vi "Dispense FN - ON - State Status (SubVI).vi"(0 "Values IN":T1 {"Drain Time (s)" format="%.2f"; "Drain Rate (g/sec)" format="%.2f"}, 1 "Settings":T2={"ON Settings"={"Enable Dynamic Setpoint?"=TRUE, "Enable Dynamic Dispense Time?"=TRUE, "Enable Drain Rate Functions"=TRUE, "Dispense Sample Time (s)"=0.5, "Dispense Slope Ave"=0, "ON Timeout (sec)"=600.0, "1st Setpoint (% of Target)"=0.0, "2nd Setpoint (% of Target)"=0.0, "3rd Setpoint (% of Target)"=0.0, "Measure Dispense Delay (sec)"=0.0, "Settle Slope Sample Time (s)"=0.0}, "OFF Settings"={"Drain Sample Time (s)"=0.5, "Drain Rate Ave Size"=5, "Drain Rate Limits (± g/sec)"=10.0, "Level Slope Range (± g/sec)"=0.25, "OFF Timeout (sec)"=0.0, "Near SP Slope Level (± g/sec)"=0.01, "Near Setpoint Threshold (%)"=95.0}, "Overshoot Settings"={"Time Limit (s)"=60.0, "Container MAX (g)"=1500.0, "Max FILL Slope (+/- g/sec)"=10.0, "% Overshot to Enable (>)"=0.25}, "FILL Timeout (s)"=300.0, "Full Settle Time (s)"=3.0, "Pre-Hydrate \nSpray Time (s)"=10.0, "Pre-Hydrate \nWait Time (s)"=30.0}, 3 "Dynamic SP Valid?":bool, 4 "Enable Dispense Measure?":bool) -> (14 "Values OUT":T1, 16 "OFF Signal":bool, 17 "Dispense Timeout?":bool, 18 "Complete":bool)   [LabVIEW 2012]
panel:
  out "Time Setpoint (Un-used)":dbl
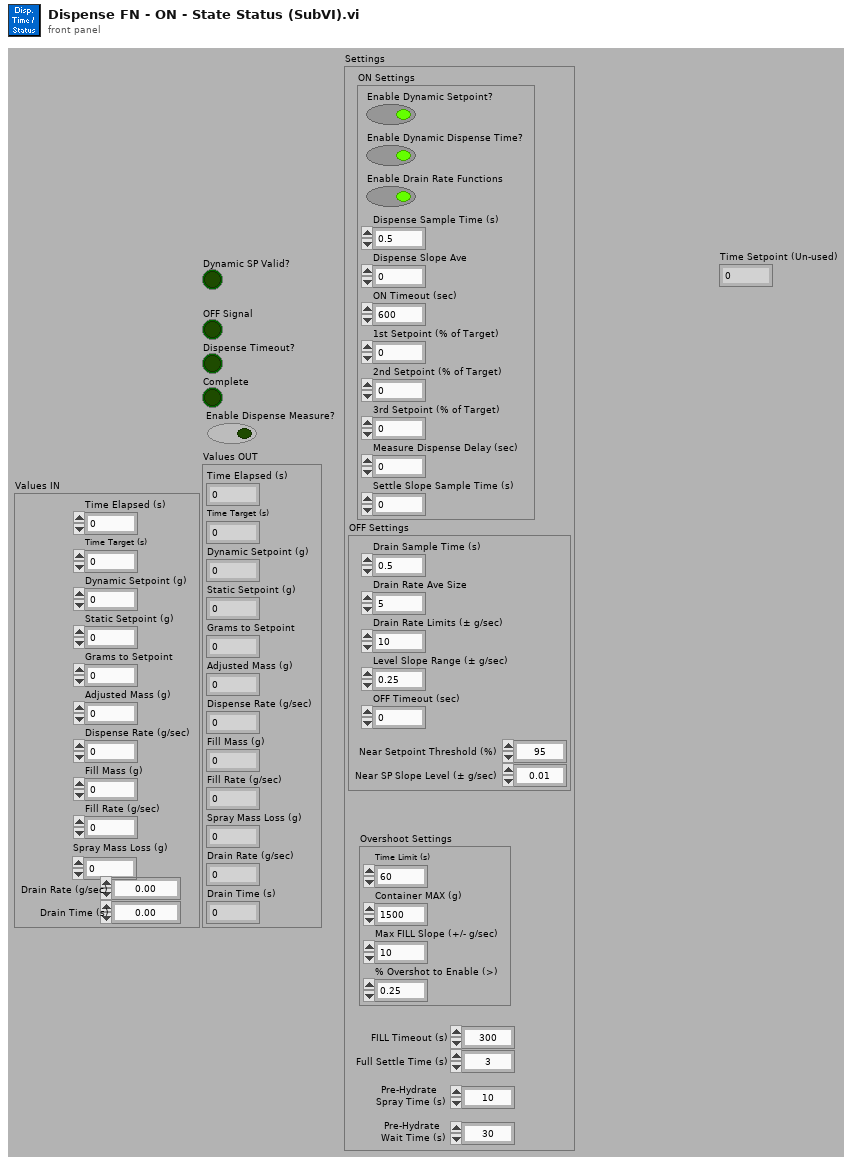
[diagram p1: front panel]
types:
  T1 = cluster{"Time Elapsed (s)":dbl, "Time Target (s)":dbl, "Dynamic Setpoint (g)":dbl, "Static Setpoint (g)":dbl, "Grams to Setpoint":dbl, "Adjusted Mass (g)":dbl, "Dispense Rate (g/sec)":dbl, "Fill Mass (g)":dbl, "Fill Rate (g/sec)":dbl, "Spray Mass Loss (g)":dbl, "Drain Rate (g/sec)":dbl, "Drain Time (s)":dbl}
  T2 = cluster{"ON Settings":cluster{"Enable Dynamic Setpoint?":bool, "Enable Dynamic Dispense Time?":bool, "Enable Drain Rate Functions":bool, "Dispense Sample Time (s)":dbl, "Dispense Slope Ave":i32, "ON Timeout (sec)":dbl, "1st Setpoint (% of Target)":dbl, "2nd Setpoint (% of Target)":dbl, "3rd Setpoint (% of Target)":dbl, "Measure Dispense Delay (sec)":dbl, "Settle Slope Sample Time (s)":dbl}, "OFF Settings":cluster{"Drain Sample Time (s)":dbl, "Drain Rate Ave Size":i32, "Drain Rate Limits (± g/sec)":dbl, "Level Slope Range (± g/sec)":dbl, "OFF Timeout (sec)":dbl, "Near SP Slope Level (± g/sec)":dbl, "Near Setpoint Threshold (%)":dbl}, "Overshoot Settings":cluster{"Time Limit (s)":dbl, "Container MAX (g)":dbl, "Max FILL Slope (+/- g/sec)":dbl, "% Overshot to Enable (>)":dbl}, "FILL Timeout (s)":dbl, "Full Settle Time (s)":dbl, "Pre-Hydrate \nSpray Time (s)":dbl, "Pre-Hydrate \nWait Time (s)":dbl}
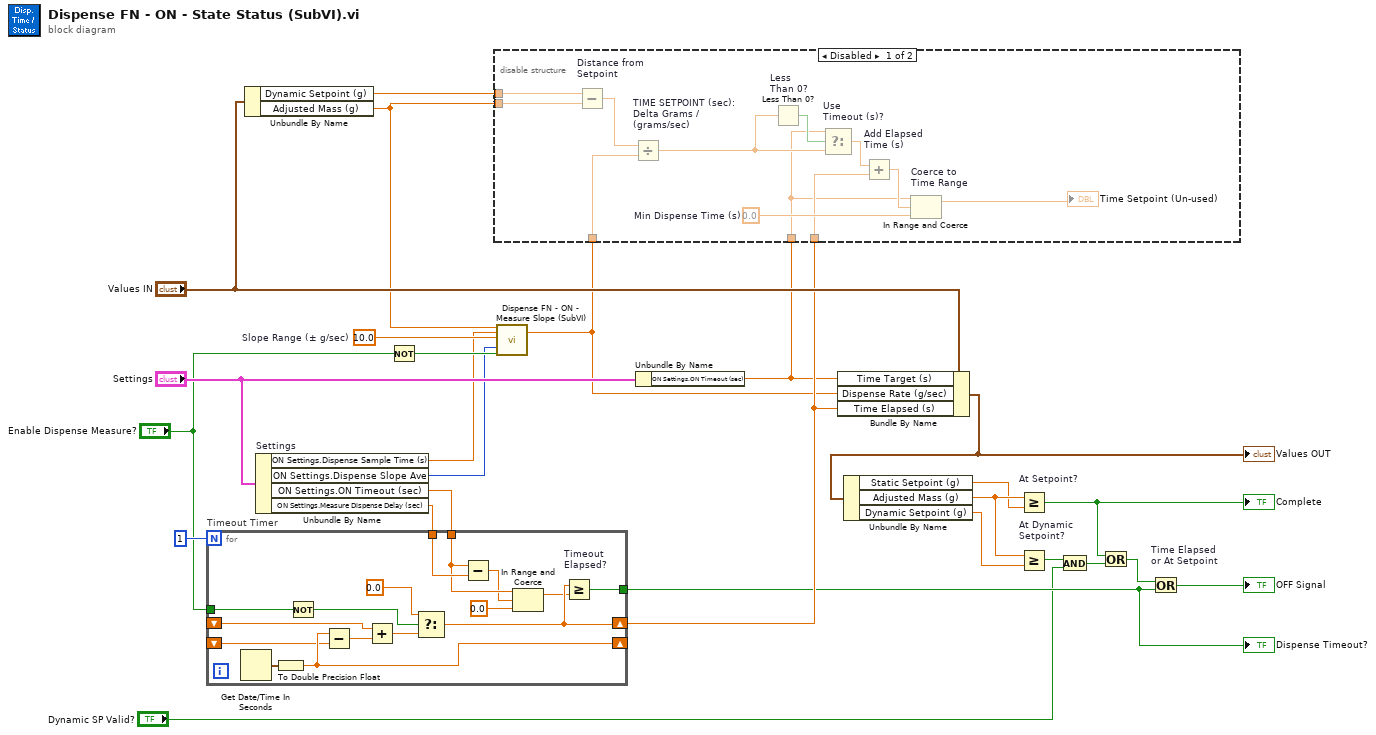
[diagram p0: block diagram]
diagram:
  w26 = 10.0  # Slope Range (± g/sec)
  n1 = Unbundle By Name("Values IN") -> ("Dynamic Setpoint (g)"=w16:dbl, "Adjusted Mass (g)"=w15:dbl)
  n2 = Unbundle By Name "Settings"("Settings") -> ("ON Settings.Dispense Sample Time (s)"=w12:dbl, "ON Settings.Dispense Slope Ave"=w11:i32, "ON Settings.ON Timeout (sec)"=w9:dbl, "ON Settings.Measure Dispense Delay (sec)"=w8:dbl)
  n3 = for "Timeout Timer" {
    N: 1 -> [_]
    shift-right: [w32] -> w17
    shift-left: _ -> [w42]
    shift-right: [w40] -> _
    shift-left: _ -> [w39]
    tunnel: [w34] -> w4
    tunnel: "Enable Dispense Measure?" -> [w37]
    tunnel: w9 -> [w30]
    tunnel: w8 -> [w31]
    n4 = Get Date/Time In Seconds() -> (seconds since 1Jan1904=w41:timestamp)
    n5 = To Double Precision Float(number=w41) -> (double precision float=w40:dbl)
    n6 = Not(x=w37) -> (.not. x?=w36:bool)
    n7 = Subtract(x=w40, y=w39) -> (x-y=w38:dbl)
    n8 = Add(x=w42, y=w38) -> (x+y=w35:dbl)
    n9 = Select(t=0.0, s=w36, f=w35) -> (s? t:f=w32:dbl)
    n10 = Subtract(x=w30, y=w31) -> (x-y=w28:dbl)
    n11 = In Range and Coerce(upper limit=w30, x=w28, lower limit=0.0) -> (coerced(x)=w27:dbl)  [unwired: 1 out]
    n12 = Greater Or Equal? "Timeout\nElapsed?"(x=w32, y=w27) -> (x >= y?=w34:bool)
  }
  "Dispense Timeout?" <- w4
  n13 = Not(x="Enable Dispense Measure?") -> (.not. x?=w14:bool)
  n14 = call "Dispense FN - ON - Measure Slope (SubVI).vi"("Measured Mass (g)"=w15, "Slope Sample Time (s)"=w12, "Slope Limits (± g/sec)"=w26, "Slope Ave Array Size"=w11, "Initialize"=w14) -> ("Ave. Slope (g/sec)"=w13:dbl)  [unwired: 1 in, 13 out]
  n15 = Unbundle By Name("Settings") -> ("ON Settings.ON Timeout (sec)"=w7:dbl)
  n16 = disable-structure shown="Disabled" {
    disable-tunnel: w17 -> [w53 _]
    disable-tunnel: w16 -> [w52 _]
    disable-tunnel: w15 -> [w46 _]
    disable-tunnel: w13 -> [w45 _]
    disable-tunnel: w7 -> [w44 _]
    frame Disabled {
      w54 = 0.0  # Min Dispense Time (s)
      n17 = Subtract "Distance from\nSetpoint"(x=w52, y=w46) -> (x-y=w51:dbl)
      n18 = Divide "TIME SETPOINT (sec):\nDelta Grams /\n(grams/sec)"(x=w51, y=w45) -> (x/y=w49:dbl)
      n19 = Less Than 0? "Less \nThan 0?"(x=w49) -> (x < 0?=w50:bool)
      n20 = Select "Use\nTimeout (s)?"(t=w44, s=w50, f=w49) -> (s? t:f=w48:dbl)
      n21 = Add "Add Elapsed\nTime (s)"(x=w48, y=w53) -> (x+y=w47:dbl)
      n22 = In Range and Coerce "Coerce to\nTime Range"(upper limit=w44, x=w47, lower limit=w54) -> (coerced(x)=→"Time Setpoint (Un-used)":dbl)  [unwired: 1 out]
    }
    frame Enabled {
    }
  }
  n23 = Bundle By Name(cluster="Values IN", "Time Target (s)"=w7, "Dispense Rate (g/sec)"=w13, "Time Elapsed (s)"=w17) -> (w19:T1)
  "Values OUT" <- w19
  n24 = Unbundle By Name(w19) -> ("Static Setpoint (g)"=w23:dbl, "Adjusted Mass (g)"=w24:dbl, "Dynamic Setpoint (g)"=w22:dbl)
  n25 = Greater Or Equal? "At Setpoint?"(x=w24, y=w23) -> (x >= y?=w6:bool)
  "Complete" <- w6
  n26 = Greater Or Equal? "At Dynamic\nSetpoint?"(x=w24, y=w22) -> (x >= y?=w3:bool)
  n27 = And(x=w3, y="Dynamic SP Valid?") -> (x .and. y?=w1:bool)
  n28 = Or(x=w6, y=w1) -> (x .or. y?=w5:bool)
  n29 = Or "Time Elapsed\nor At Setpoint"(x=w5, y=w4) -> (x .or. y?=→"OFF Signal":bool)
